vi "Read Test Manager.vi"(8 "error in (no error)":errorcluster, 10 "VI Call Chain":string[](array[string]), 11 "Assert Factory in":refnum<class "Test Assert Factory.lvclass">) -> (0 "error out":errorcluster, 2 "Test Manager":refnum<class "Test Manager.lvclass">, 3 "Assert Factory out":refnum<class "Test Assert Factory.lvclass">)   [LabVIEW 2009, in "Caraya.lvlib" / "Test Assert Factory.lvclass"]
doc: "Returns the Test Manager implementation being used for a specific VI."
uses:
  Test Assert Factory.lvclass
  Basic Test Manager/Basic Test Manager.lvclass
  Test Manager/Test Manager.lvclass
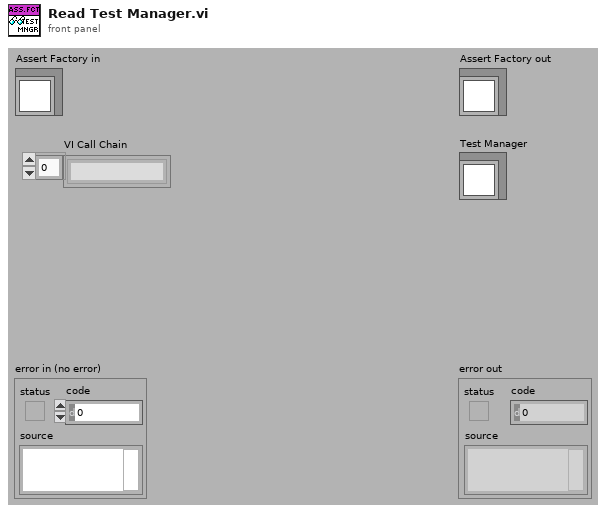
[diagram p1: front panel]
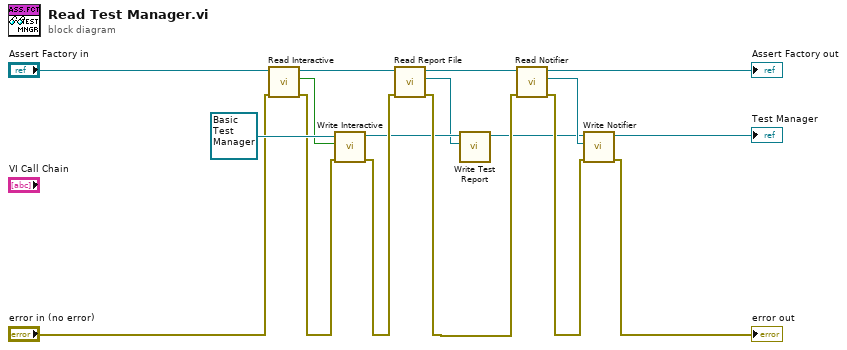
[diagram p0: block diagram]
diagram:
  n1 = call "Read Interactive.vi"("error in (no error)"="error in (no error)", "Test Assert Factory in"="Assert Factory in") -> ("error out"=w11:errorcluster, "Interactive"=w15:bool, "Test Assert Factory out"=w14:refnum<class "Test Assert Factory.lvclass">)  [unwired: 7 in]
  n2 = call "Write Interactive.vi"("error in (no error)"=w11, "Interactive"=w15, "Basic Test Manager in"=refnum<class "Basic Test Manager.lvclass"> refnum ("Caraya.lvlib:Basic Test Manager.lvclass")) -> ("error out"=w13:errorcluster, "Basic Test Manager out"=w3:refnum<class "Basic Test Manager.lvclass">)  [unwired: 7 in]
  n3 = call "Read Report File.vi"("error in (no error)"=w13, "Test Assert Factory in"=w14) -> ("error out"=w4:errorcluster, "Test Report"=w2:refnum<class "Test Report.lvclass">, "Test Assert Factory out"=w10:refnum<class "Test Assert Factory.lvclass">)  [unwired: 7 in]
  n4 = call "Write Test Report.vi"("Test Report"=w2, "Test Manager in"=w3) -> ("Test Manager out"=w1:refnum<class "Basic Test Manager.lvclass">)  [unwired: 9 in]
  n5 = call "Read Notifier.vi"("error in (no error)"=w4, "Test Assert Factory in"=w10) -> ("error out"=w8:errorcluster, "notifier"=w6:refnum<notifier>, "Test Assert Factory out"=→"Assert Factory out":refnum<class "Test Assert Factory.lvclass">)  [unwired: 7 in]
  n6 = call "Write Notifier.vi"("error in (no error)"=w8, "notifier"=w6, "Basic Test Manager in"=w1) -> ("error out"=→"error out":errorcluster, "Basic Test Manager out"=→"Test Manager":refnum<class "Basic Test Manager.lvclass">)  [unwired: 7 in]
